vi "Initialize Sessions.vi"(0 "Session Handle in":T1, 11 "error in (no error)":errorcluster) -> (4 "Session Handle out":T1, 15 "error out":errorcluster)   [LabVIEW 2015, in "Environics.lvclass"]
uses:
  Environics.lvclass
  Typedefs/Session Handle.ctl
  C:/TMflex/Test Fixtures/PAS Calibration/Distributed/EnvComm.dll
  EnvComm.dll
  Environics.lvclass/Environics.ctl
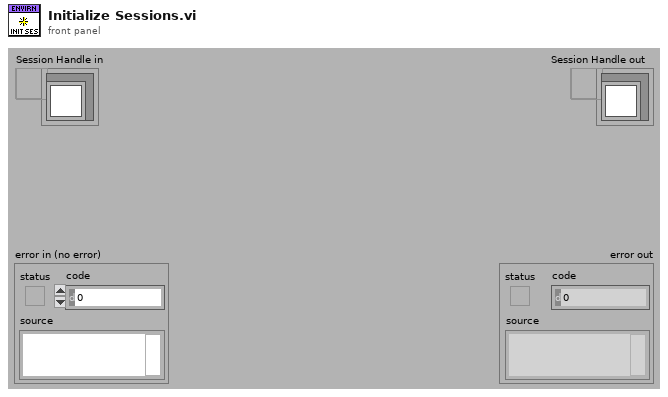
[diagram p1: front panel]
types:
  T1 = typedef "Environics.lvclass/Session Handle.ctl" = refnum<data-value>
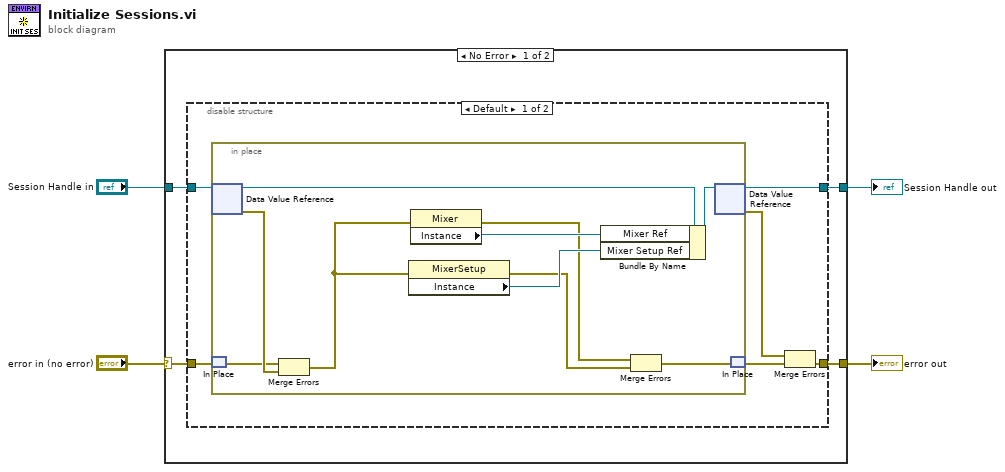
[diagram p0: block diagram]
diagram:
  n1 = case shown="No Error" "error in (no error)" {
    selector: "error in (no error)" -> [w5 w27]
    tunnel: "Session Handle in" -> [w8 w28]
    tunnel: [w7 w28] -> w3
    tunnel: [w6 w27] -> w2
    frame No Error {
      n2 = disable-structure shown="Default" {
        disable-tunnel: w8 -> [w14 w26]
        disable-tunnel: [w13 w26] -> w7
        disable-tunnel: [w12 w25] -> w6
        disable-tunnel: w5 -> [w11 w25]
        frame condition #0 (active) {
          n3 = in-place {
            n4 = in-place-dvr #1(w14) -> (w22:refnum<class "Environics.lvclass">, w24:errorcluster)
            n5 = in-place-match #2(w11) -> (w23:errorcluster)
            n6 = Merge Errors(w23, w24) -> (w15:errorcluster)
            n7 = property class="MixerSetup"(error in=w15) -> (error out=w16:errorcluster, "Instance"=w18:refnum<k24>)  [unwired: 1 in, 1 out]
            n8 = property class="Mixer"(error in=w15) -> (error out=w17:errorcluster, "Instance"=w19:refnum<k24>)  [unwired: 1 in, 1 out]
            n9 = Bundle By Name(cluster=w22, "Mixer Ref"=w19, "Mixer Setup Ref"=w18) -> (w21:refnum<class "Environics.lvclass">)
            n10 = Merge Errors(w17, w16) -> (w20:errorcluster)
            n11 = in-place-dvr #1(w21) -> (w13:T1, w9:errorcluster)
            n12 = in-place-match #2(w20) -> (w10:errorcluster)
          }
          n13 = Merge Errors(w9, w10) -> (w12:errorcluster)
        }
        frame condition #1 {
        }
      }
    }
    frame Error {
    }
  }
  "Session Handle out" <- w3
  "error out" <- w2
